vi "Control - GDI - Load Command.vi"(11 "Control Inputs":T1={"Engine Speed [RPM]"=0.0, "Engine Status"=enum."STALLED", "Load Control \nMode"=enum."No Governor", "MAX_CAT"=0, "dt(s)"=0.0, "Sync Stopped"=FALSE, "Number of Cylinders"=0, "Engine Displacement [cc]"=0.0, "StoichAFR"=0.0, "Q.LHV Fuel [kJ/kg]"=0.0, "BattV PSU [V]"=0.0, "12V PSU [V]"=0.0, "5V PSU [V]"=0.0, "Pedal Position [%]"=0.0, "Oil Pressure [kPa]"=0.0, "Oil Temp [C]"=0.0, "Oil Level [%]"=0.0, "Engine Coolant Temp (ECT) [C]"=0.0, "Engine Coolant Pressure [kPa]"=0.0, "Rail Pressure [bar]"=0.0, "Fuel Pressure [kPa]"=0.0, "Fuel Temp [C]"=0.0, "Vacuum Pressure [kPa]"=0.0, "Throttle Position [%]"=0.0, "Cam1 Advance [CAD]"=0.0, "Cam2 Advance [CAD]"=0.0, "CA50 Control Output [CAD]"=[], "CA50 Control Output Valid"=[], "Oil Level Switch"=FALSE, "Intake Air Temp (IAT) [C]"=0.0, "Barometric Air Pressure [kPa]"=0.0, "Intake Air Rel. Humidity [%]"=0.0, "Mass Air Flow (MAF) [kg/hr]"=0.0, "Turbo Inlet Air Pressure [kPa]"=0.0, "Turbo Inlet Air Temp [C]"=0.0, "Turbo Outlet Air Pressure [kPa]"=0.0, "Turbo Outlet Air Temp [C]"=0.0, "CAC Outlet Pressure [kPa]"=0.0, "CAC Outlet Temp [C]"=0.0, "Intake Manifold Pressure (MAP) [kPa]"=0.0, "Intake Manifold Temp (MAT) [C]"=0.0, "Exhaust Manifold Pressure [kPa]"=0.0, "Exhaust Manifold Temp [C]"=0.0, "HighP EGR Cooler Outlet Pressure [kPa]"=0.0, "HighP EGR Cooler Outlet Temp [C]"=0.0, "HighP EGR Differential Pressure [kPa]"=0.0, "HighP EGR Valve Position [%]"=0.0, "Turbo Outlet Exhaust Pressure [kPa]"=0.0, "Turbo Outlet Exhaust Temp [C]"=0.0, "VGT Position 1 [%]"=0.0, "VGT Position 2 [%]"=0.0, "Turbo Speed 1 [RPM]"=0.0, "Turbo Speed 2 [RPM]"=0.0, "LowP EGR Differential Pressure [kPa]"=0.0, "LowP EGR Valve Position [%]"=0.0, "UEGO1Lambda"=0.0, "UEGO1_Hot"=FALSE, "UEGO2Lambda"=0.0, "UEGO2_Hot"=FALSE} {"CA50 Control Output [CAD]" format="%.2f"; "VGT Position 1 [%]" format="%.2f"; "Turbo Speed 2 [RPM]" format="%.2f"; "LowP EGR Valve Position [%]" format="%.2f"; "Turbo Outlet Exhaust Temp [C]" format="%.2f"; "Barometric Air Pressure [kPa]" format="%#_6f"; "UEGO2Lambda" format="%.2f"; "HighP EGR Valve Position [%]" format="%.2f"; "HighP EGR Differential Pressure [kPa]" format="%.2f"; "Turbo Speed 1 [RPM]" format="%.2f"; "UEGO1Lambda" format="%.2f"; "Mass Air Flow (MAF) [kg/hr]" format="%#_6f"}) -> (1 "Integral Governor Control [%]":sgl, 2 "Rapid (P+D) Governor Control [%]":sgl, 3 "IMEP Desired [bar]":sgl)   [LabVIEW 2015, in "ECS-RT.lvlib"]
uses:
  ECS-RT.lvlib
  Typedefs/MISC/Load Control Mode.ctl
  ECS-Shared.lvlib
  Typedefs/Control Inputs/Control Inputs.ctl
  Typedefs/EPT/Engine Status.ctl
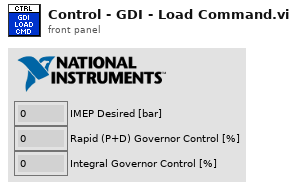
[diagram p1: front panel]
types:
  T1 = typedef "ECS-Shared.lvlib/Control Inputs.ctl" = cluster{"Engine Speed [RPM]":sgl, "Engine Status":T2, "Load Control \nMode":T3, "MAX_CAT":u16, "dt(s)":sgl, "Sync Stopped":bool, "Number of Cylinders":u8, "Engine Displacement [cc]":sgl, "StoichAFR":sgl, "Q.LHV Fuel [kJ/kg]":sgl, "BattV PSU [V]":sgl, "12V PSU [V]":sgl, "5V PSU [V]":sgl, "Pedal Position [%]":sgl, "Oil Pressure [kPa]":sgl, "Oil Temp [C]":sgl, "Oil Level [%]":sgl, "Engine Coolant Temp (ECT) [C]":sgl, "Engine Coolant Pressure [kPa]":sgl, "Rail Pressure [bar]":sgl, "Fuel Pressure [kPa]":sgl, "Fuel Temp [C]":sgl, "Vacuum Pressure [kPa]":sgl, "Throttle Position [%]":sgl, "Cam1 Advance [CAD]":sgl, "Cam2 Advance [CAD]":sgl, "CA50 Control Output [CAD]":sgl[], "CA50 Control Output Valid":bool[], "Oil Level Switch":bool, "Intake Air Temp (IAT) [C]":sgl, "Barometric Air Pressure [kPa]":sgl, "Intake Air Rel. Humidity [%]":sgl, "Mass Air Flow (MAF) [kg/hr]":sgl, "Turbo Inlet Air Pressure [kPa]":sgl, "Turbo Inlet Air Temp [C]":sgl, "Turbo Outlet Air Pressure [kPa]":sgl, "Turbo Outlet Air Temp [C]":sgl, "CAC Outlet Pressure [kPa]":sgl, "CAC Outlet Temp [C]":sgl, "Intake Manifold Pressure (MAP) [kPa]":sgl, "Intake Manifold Temp (MAT) [C]":sgl, "Exhaust Manifold Pressure [kPa]":sgl, "Exhaust Manifold Temp [C]":sgl, "HighP EGR Cooler Outlet Pressure [kPa]":sgl, "HighP EGR Cooler Outlet Temp [C]":sgl, "HighP EGR Differential Pressure [kPa]":sgl, "HighP EGR Valve Position [%]":sgl, "Turbo Outlet Exhaust Pressure [kPa]":sgl, "Turbo Outlet Exhaust Temp [C]":sgl, "VGT Position 1 [%]":sgl, "VGT Position 2 [%]":sgl, "Turbo Speed 1 [RPM]":sgl, "Turbo Speed 2 [RPM]":sgl, "LowP EGR Differential Pressure [kPa]":sgl, "LowP EGR Valve Position [%]":sgl, "UEGO1Lambda":sgl, "UEGO1_Hot":bool, "UEGO2Lambda":sgl, "UEGO2_Hot":bool}
  T2 = typedef "ECS-Shared.lvlib/Engine Status.ctl" = enum16{"OFF", "STALLED", "CRANKING", "RUNNING", "ACCEL", "DECEL", "SAFE"}
  T3 = typedef "ECS-Shared.lvlib/Load Control Mode.ctl" = enum16{"No Governor", "Low-Idle Governor", "Max Speed Governor"}
  T4 = typedef "ECS-Shared.lvlib/Control Inputs.ctl" = cluster{"Engine Speed [RPM]":sgl, "Engine Status":T2, "Load Control \nMode":T3, "dt(s)":sgl, "Number of Cylinders":u8, "Engine Displacement [cc]":sgl, "StoichAFR":sgl, "Q.LHV Fuel [kJ/kg]":sgl, "BattV PSU [V]":sgl, "12V PSU [V]":sgl, "5V PSU [V]":sgl, "Pedal Position [%]":sgl, "Oil Pressure [kPa]":sgl, "Oil Temp [C]":sgl, "Oil Level [%]":sgl, "Engine Coolant Temp (ECT) [C]":sgl, "Engine Coolant Pressure [kPa]":sgl, "Rail Pressure [bar]":sgl, "Fuel Pressure [kPa]":sgl, "Fuel Temp [C]":sgl, "Vacuum Pressure [kPa]":sgl, "Throttle Position [%]":sgl, "Cam1 Advance [CAD]":sgl, "Cam2 Advance [CAD]":sgl, "Cam3 Advance [CAD]":sgl, "Cam4 Advance [CAD]":sgl, "CA50 Control Output [CAD]":sgl[], "CA50 Control Output Valid":bool[], "Intake Air Temp (IAT) [C]":sgl, "Barometric Air Pressure [kPa]":sgl, "Intake Air Rel. Humidity [%]":sgl, "Mass Air Flow (MAF) [kg/hr]":sgl, "Turbo Inlet Air Pressure [kPa]":sgl, "Turbo Inlet Air Temp [C]":sgl, "Turbo Outlet Air Pressure [kPa]":sgl, "Turbo Outlet Air Temp [C]":sgl, "CAC Outlet Pressure [kPa]":sgl, "CAC Outlet Temp [C]":sgl, "Intake Manifold Pressure (MAP) [kPa]":sgl, "Intake Manifold Temp (MAT) [C]":sgl, "Exhaust Manifold Pressure [kPa]":sgl, "Exhaust Manifold Temp [C]":sgl, "HighP EGR Cooler Outlet Pressure [kPa]":sgl, "HighP EGR Cooler Outlet Temp [C]":sgl, "HighP EGR Differential Pressure [kPa]":sgl, "HighP EGR Valve Position [%]":sgl, "Turbo Outlet Exhaust Pressure [kPa]":sgl, "Turbo Outlet Exhaust Temp [C]":sgl, "VGT Position 1 [%]":sgl, "VGT Position 2 [%]":sgl, "Turbo Speed 1 [RPM]":sgl, "Turbo Speed 2 [RPM]":sgl, "LowP EGR Differential Pressure [kPa]":sgl, "LowP EGR Valve Position [%]":sgl, "UEGO1Lambda":sgl, "UEGO1_Hot":bool, "UEGO2Lambda":sgl, "UEGO2_Hot":bool, "Knock Intensity":sgl[], "Knock":bool[]}
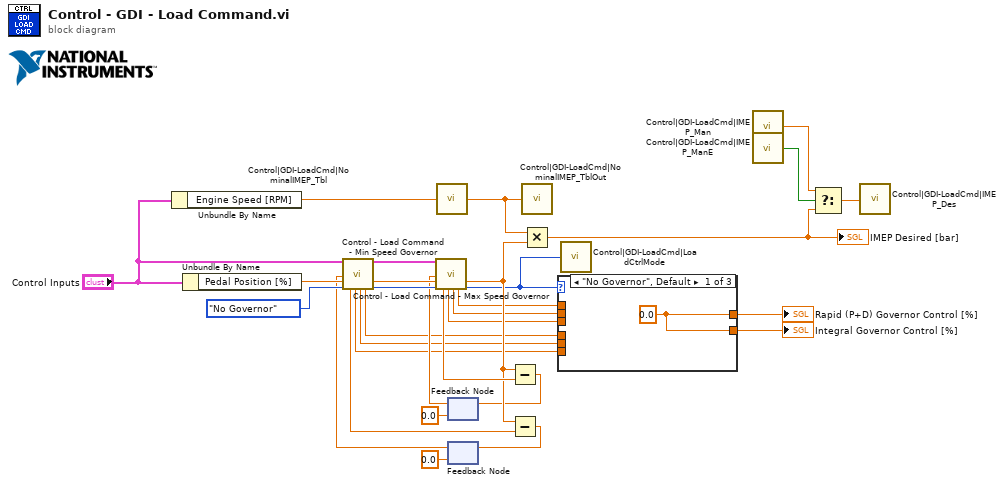
[diagram p0: block diagram]
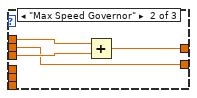
[diagram p2: hidden frame]
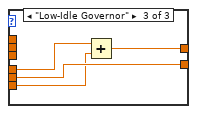
[diagram p3: hidden frame]
diagram:
  n1 = Unbundle By Name("Control Inputs") -> ("Engine Speed [RPM]"=w30:sgl)
  n2 = Unbundle By Name("Control Inputs") -> ("Pedal Position [%]"=w27:sgl)
  n3 = call "Control|GDI-LoadCmd|NominalIMEP_Tbl"("X Index"=w30) -> ("Y"=w29:sgl)
  n4 = feedback #1(sgl 0.0) -> (w18:sgl)
  n5 = feedback #2(sgl 0.0) -> (w16:sgl)
  n6 = call "Control - Load Command - Min Speed Governor.vi"("Control Inputs"="Control Inputs", "BeatbackDiff"=w16, "Pedal In"=w27, "Load Control Mode In"=Load_Control_Mode."No Governor") -> ("Governor Output"=w20:sgl, "PEffort"=w10:sgl, "IEffort"=w11:sgl, "DEffort"=w12:sgl, "Control Inputs"=w23:T4, "Pedal Out"=w26:sgl, "Load Control Mode Out"=w25:T3)  [unwired: 9 in]
  n7 = call "Control - Load Command - Max Speed Governor.vi"("Control Inputs"=w23, "BeatbackDiff"=w18, "Pedal In"=w26, "Load Control Mode In"=w25) -> ("Governor Output"=w22:sgl, "PEffort"=w13:sgl, "IEffort"=w14:sgl, "DEffort"=w15:sgl, "Pedal Out"=w21:sgl, "Load Control Mode Out"=w3:T3)  [unwired: 9 in, 1 out]
  n8 = Subtract(x=w21, y=w22) -> (x-y=w19:sgl)
  n9 = feedback-in #1(w19) -> ()
  n10 = Subtract(x=w21, y=w20) -> (x-y=w17:sgl)
  n11 = feedback-in #2(w17) -> ()
  n12 = call "Control|GDI-LoadCmd|NominalIMEP_TblOut"("Value"=w29) -> ()
  n13 = Multiply(x=w29, y=w21) -> (x*y=w5:sgl)
  "IMEP Desired [bar]" <- w5
  n14 = case shown="\"No Governor\", Default" w3 {
    tunnel: w15 -> [_ w35 _]
    tunnel: w14 -> [_ w32 _]
    tunnel: w13 -> [_ w34 _]
    tunnel: w12 -> [_ _ w36]
    tunnel: w11 -> [_ _ w38]
    tunnel: w10 -> [_ _ w37]
    tunnel: [w31 w33 w39] -> w9
    tunnel: [w31 w32 w38] -> w8
    frame "No Governor", Default {
      w31 = sgl 0.0 ("Rapid (P+D) Governor Control")
    }
    frame "Max Speed Governor" {
      n15 = Add(x=w35, y=w34) -> (x+y=w33:sgl)
    }
    frame "Low-Idle Governor" {
      n16 = Add(x=w36, y=w37) -> (x+y=w39:sgl)
    }
  }
  "Rapid (P+D) Governor Control [%]" <- w9
  "Integral Governor Control [%]" <- w8
  n17 = call "Control|GDI-LoadCmd|LoadCtrlMode"("Value"=w3) -> ()
  n18 = call "Control|GDI-LoadCmd|IMEP_Man"() -> ("Value"=w7:sgl)
  n19 = call "Control|GDI-LoadCmd|IMEP_ManE"() -> ("Value"=w6:bool)
  n20 = Select(t=w7, s=w6, f=w5) -> (s? t:f=w4:sgl)
  n21 = call "Control|GDI-LoadCmd|IMEP_Des"("Value"=w4) -> ()
